vi "Day10-02_패턴 매칭.vi"() -> ()   [LabVIEW 2021]
uses:
  <vilib>/vision/NI_Vision_Development_Module.lvlib
panel:
  out "Matches":T1(array[cluster]) {"Bounding Box"."y" format="%.2f"; "Bounding Box"."x" format="%.2f"; "Position"."y" format="%.2f"; "Position"."x" format="%.2f"; "Score" format="%.2f"; "Scale" format="%.2f"; "Angle" format="%.2f"}
  out "Image":T2(plugin-control)
  out "템플릿":T2(plugin-control)
  in  "템플릿 저장경로":path
  in  "템플릿 생성":bool
  in  "판별":bool
  in  "정지":bool
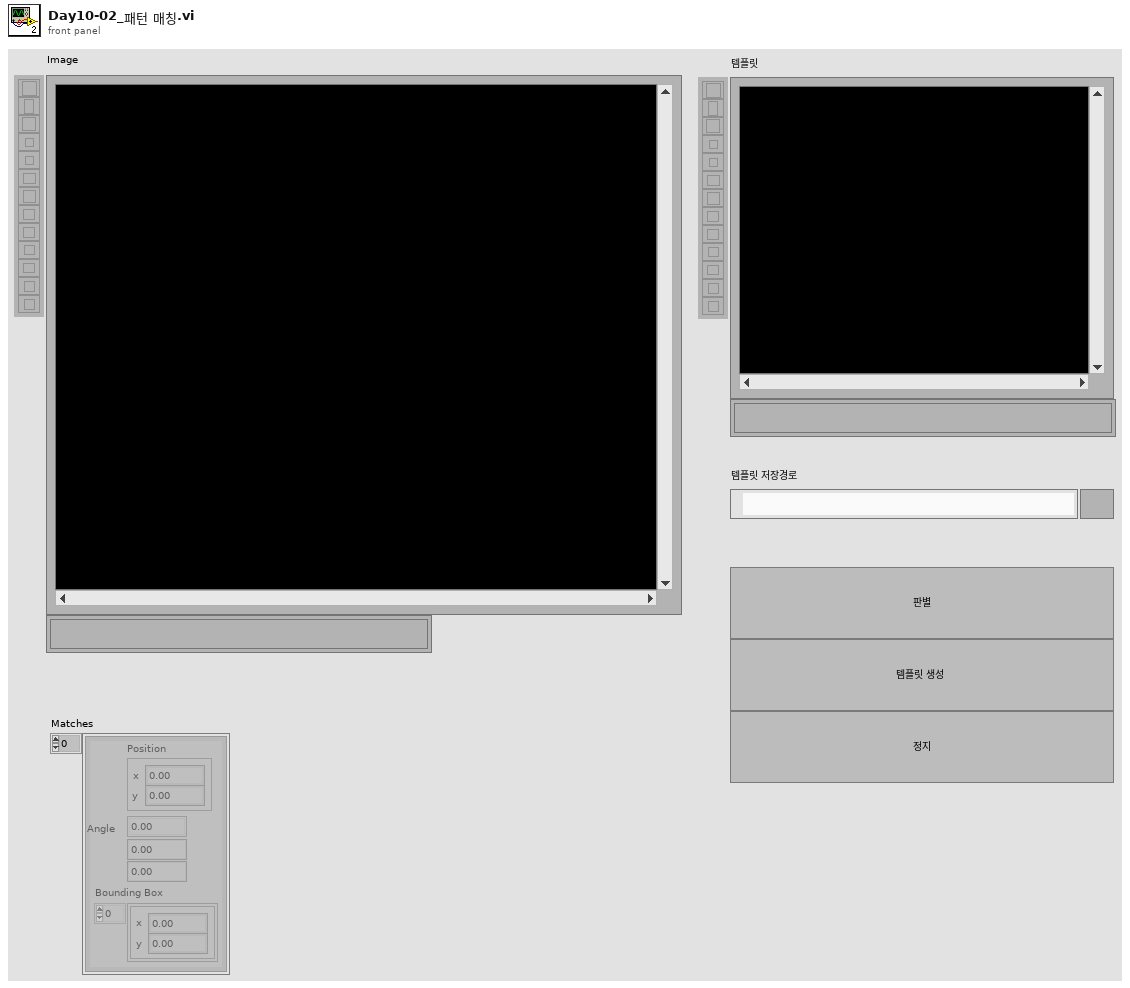
[diagram p1: front panel]
types:
  T1 = cluster{"Position":cluster{"x":sgl, "y":sgl}, "Angle":sgl, "Scale":sgl, "Score":sgl, "Bounding Box":cluster{"x":sgl, "y":sgl}[]}[]
  T2 = typedef "IMAQ Image.ctl" = refnum<image>
  T3 = typedef "Image Type" = u32
  T4 = typedef "ROI Descriptor" = cluster{"Global Rectangle":i32[], "Contours":cluster{"ID":enum32{"External", "Internal"}, "Type":u32, "Coordinates":i32[]}[]}
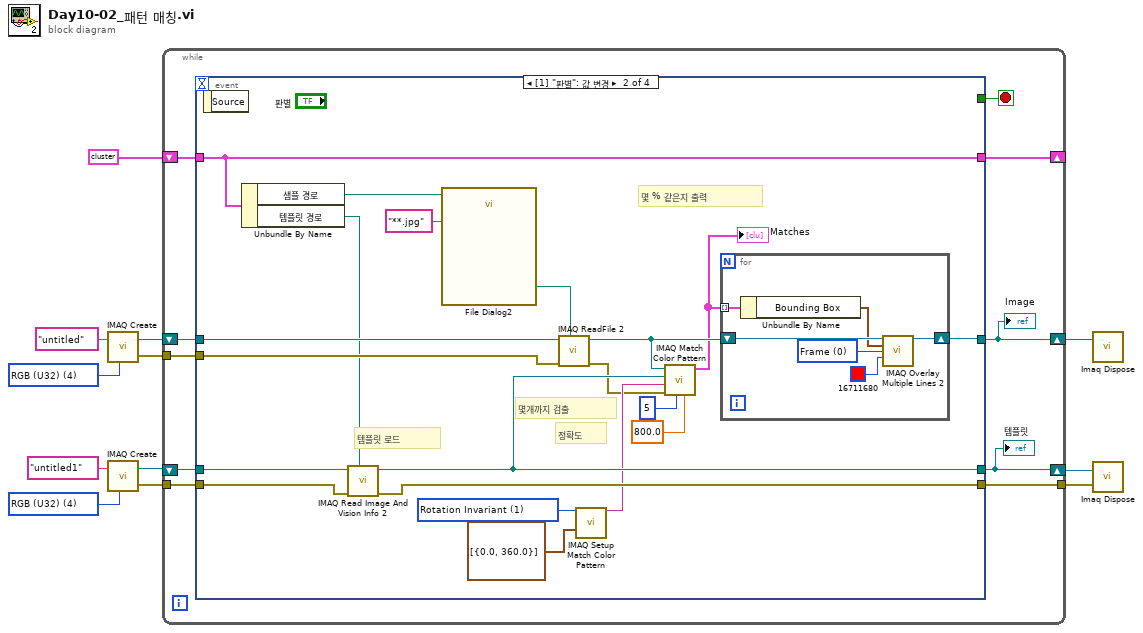
[diagram p0: block diagram]
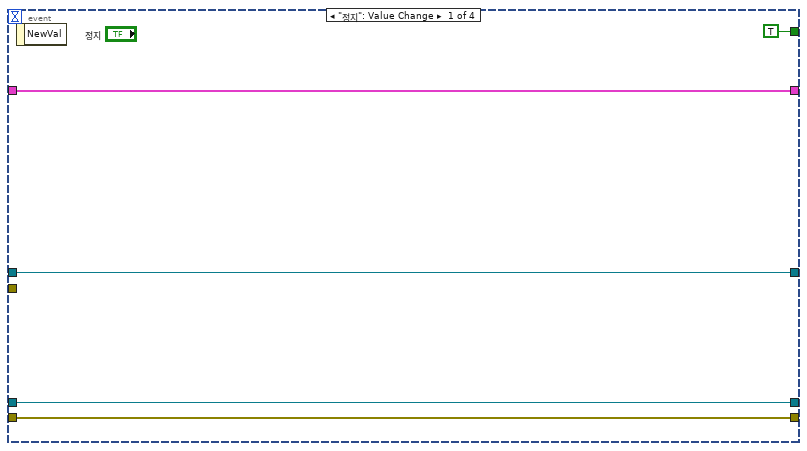
[diagram p2: hidden frame]
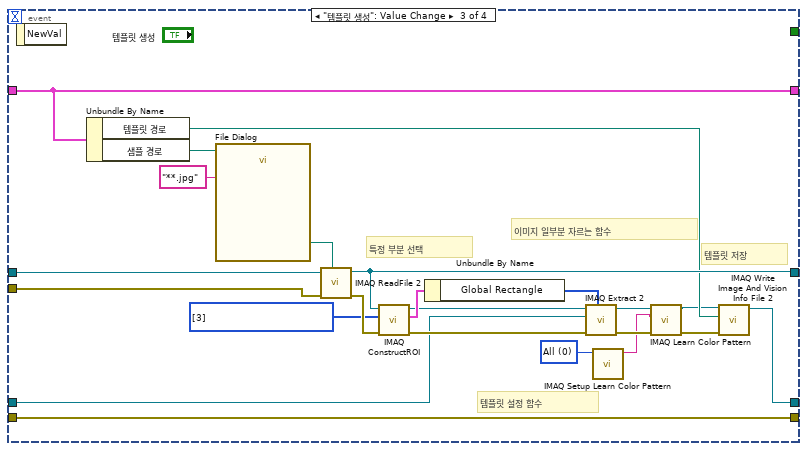
[diagram p3: hidden frame]
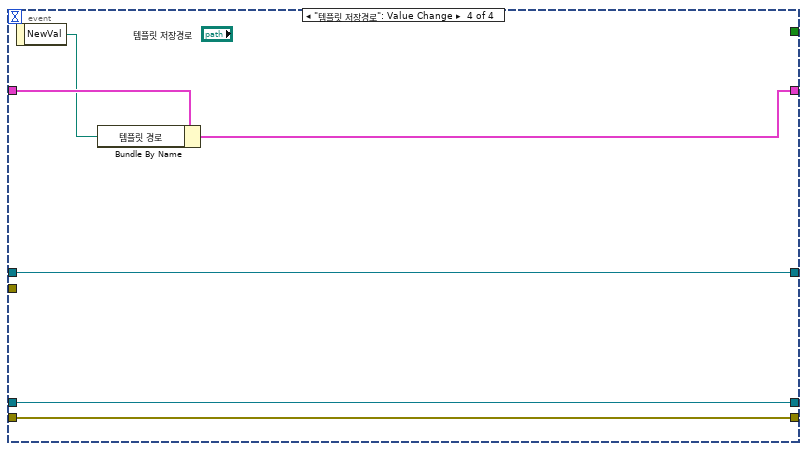
[diagram p4: hidden frame]
diagram:
  w6 = T3 4 items=["Grayscale (U8)", "Grayscale (I16)", "Grayscale (SGL)", "Complex (CSG)", "RGB (U32)", "HSL (U32)", "RGB (U64)", "Grayscale (U16)"] ("Image Type")
  w10 = T3 4 items=["Grayscale (U8)", "Grayscale (I16)", "Grayscale (SGL)", "Complex (CSG)", "RGB (U32)", "HSL (U32)", "RGB (U64)", "Grayscale (U16)"] ("Image Type")
  n1 = call "IMAQ Create"("Image Name"="untitled", "Image Type"=w10) -> ("New Image"=w12:T2, "error out"=w11:errorcluster)  [unwired: 2 in, 1 out]
  n2 = call "IMAQ Create"("Image Name"="untitled1", "Image Type"=w6) -> ("New Image"=w8:T2, "error out"=w7:errorcluster)  [unwired: 2 in, 1 out]
  n3 = while {
    shift-right: [w18] -> _
    shift-left: cluster{"샘플 경로":path, "템플릿 경로":path} {"샘플 경로"=path "C:/Embedded_System/04_LabVIEW/Programming_SourceCode/LabVIEW/이미지파일", "템플릿 경로"=path "C:/Embedded_System/04_LabVIEW/Programming_SourceCode/LabVIEW/Day10_0412/탬플릿1.png"} -> [w19]
    shift-right: [w14] -> w3
    shift-left: w12 -> [w20]
    shift-right: [w13] -> w2
    shift-left: w8 -> [w17]
    tunnel: w11 -> [w22]
    tunnel: w7 -> [w21]
    tunnel: [w15] -> w1
    stop <- w16 stop-if-true
    n4 = event shown="[1] \"판별\": 값 변경" {
      selector: _ -> [_ _ _ _]
      dyn-events: _ -> [_ _ _ _]
      timeout: _ -> [_ _ _ _]
      tunnel: w22 -> [_ w42 w72 _]
      tunnel: w21 -> [w25 w39 w61 w77]
      tunnel: w20 -> [w27 w43 w75 w79]
      tunnel: [w27 w41 w69 w79] -> w14
      tunnel: w19 -> [w26 w47 w76 w82]
      tunnel: [w26 w47 w76 w80] -> w18
      tunnel: [w25 w38 w61 w77] -> w15
      tunnel: [w24 w36 w63 w78] -> w13
      tunnel: w17 -> [w24 w40 w65 w78]
      tunnel: [TRUE _ _ _] -> w16
      event "정지": Value Change {
        n5 = event-data() -> ()  [unwired: 1 in, 1 out]
      }
      event "판별": Value Change {
        w32 = u32 1 items=["Shift Invariant", "Rotation Invariant"] ("Match Mode")
        # "몇 % 같은지 출력"
        # "템플릿 로드"
        # "몇개까지 검출"
        # "정확도"
        n6 = event-data() -> ()  [unwired: 1 in, 1 out]
        n7 = Unbundle By Name(w47) -> ("샘플 경로"=w46:path, "템플릿 경로"=w37:path)
        n8 = call "IMAQ Read Image And Vision Info 2"("File Path"=w37, "error in (no error)"=w39, "Image"=w40) -> ("error out"=w38:errorcluster, "Image Out"=w36:T2)  [unwired: 6 in, 1 out]
        n9 = call "File Dialog2"("start path"=w46, "pattern (all files)"="**.jpg") -> ("selected path"=w44:path)  [unwired: 5 in, 8 out]
        n10 = call "IMAQ ReadFile 2"("File Path"=w44, "error in (no error)"=w42, "Image"=w43) -> ("error out"=w29:errorcluster, "Image Out"=w30:T2)  [unwired: 4 in, 3 out]
        n11 = call "IMAQ Setup Match Color Pattern"("Match Mode"=w32, "Rotation Angle Ranges (degrees)"=cluster{sgl, sgl}[] [{0.0, 360.0}]) -> ("Match Color Pattern Setup Data"=w33:string)  [unwired: 12 in, 1 out]
        n12 = call "IMAQ Match Color Pattern"("Minimum Match Score"=sgl 800.0, "Number of Matches Requested"=5, "error in (no error)"=w29, "Match Color Pattern Setup Data"=w33, "Template Image"=w36, "Image"=w30) -> ("Matches"=w28:T1)  [unwired: 3 in, 2 out]
        "Matches" <- w28
        n13 = for {
          shift-right: [w52] -> w41
          shift-left: w30 -> [w53]
          tunnel: w28 -> [w51] mode=indexing
          w49 = u32 0 items=["Frame", "Fill"] ("Drawing Mode (Frame)")
          n14 = Unbundle By Name(w51) -> ("Bounding Box"=w50:cluster{"x":sgl, "y":sgl}[])
          n15 = call "IMAQ Overlay Multiple Lines 2"("Image"=w53, "Line End Points"=w50, "Drawing Mode (Frame)"=w49, "Color"=u32 16711680) -> ("Image Out"=w52:T2)  [unwired: 10 in, 1 out]
        }
      }
      event "템플릿 생성": Value Change {
        w54 = u32 0 items=["All", "Shift Information", "Rotation Information"] ("Learn Mode")
        w62 = u32[] [3] items=["No Selection", "Point", "Line", "Rectangle", "Oval", "Polygon", "Freehand Region", "Annulus", "Zoom", "Pan", "Broken Line", "Freehand Line", "Rotated Rectangle"] ("Tools")
        # "템플릿 설정 함수"
        # "템플릿 저장"
        # "특정 부분 선택"
        # "이미지 일부분 자르는 함수"
        n16 = event-data() -> ()  [unwired: 1 in, 1 out]
        n17 = Unbundle By Name(w76) -> ("템플릿 경로"=w64:path, "샘플 경로"=w74:path)
        n18 = call "File Dialog"("start path"=w74, "pattern (all files)"="**.jpg") -> ("selected path"=w73:path)  [unwired: 5 in, 8 out]
        n19 = call "IMAQ ReadFile 2"("File Path"=w73, "error in (no error)"=w72, "Image"=w75) -> ("error out"=w71:errorcluster, "Image Out"=w69:T2)  [unwired: 4 in, 3 out]
        n20 = call "IMAQ ConstructROI"("error in (no error)"=w71, "Tools"=w62, "Image"=w69) -> ("error out"=w67:errorcluster, "ROI Descriptor Out"=w70:T4, "Image Out (duplicate)"=w68:T2)  [unwired: 5 in, 1 out]
        n21 = Unbundle By Name(w70) -> ("Global Rectangle"=w66:i32[])
        n22 = call "IMAQ Extract 2"("Optional Rectangle"=w66, "error in (no error)"=w67, "Image Dst"=w65, "Image Src"=w68) -> ("error out"=w57:errorcluster, "Image Dst Out"=w59:T2)  [unwired: 6 in]
        n23 = call "IMAQ Setup Learn Color Pattern"("Learn Mode"=w54) -> ("Learn Color Pattern Setup Data"=w55:string)  [unwired: 9 in, 1 out]
        n24 = call "IMAQ Learn Color Pattern"("error in (no error)"=w57, "Learn Color Pattern Setup Data"=w55, "Image"=w59) -> ("error out"=w56:errorcluster, "Template Image Out"=w58:T2)  [unwired: 7 in]
        n25 = call "IMAQ Write Image And Vision Info File 2"("error in (no error)"=w56, "File Path"=w64, "Image"=w58) -> ("Image Out (duplicate)"=w63:T2)  [unwired: 7 in, 1 out]
      }
      event "템플릿 저장경로": Value Change {
        n26 = event-data() -> ("NewVal"=w81:path)  [unwired: 1 in]
        n27 = Bundle By Name(cluster=w82, "템플릿 경로"=w81) -> (w80:cluster{"샘플 경로":path, "템플릿 경로":path})
      }
    }
    "템플릿" <- w13
    "Image" <- w14
  }
  n28 = call "Imaq Dispose"("Image"=w3) -> ()  [unwired: 5 in, 1 out]
  n29 = call "Imaq Dispose"("Image"=w2, "error in (no error)"=w1) -> ()  [unwired: 4 in, 1 out]
